vi "Callback_Roller_Fire.vi"   [LabVIEW 2011]
uses:
  roller/roller_internal_state.ctl
  roller/roller_globals.vi
types:
  T1 = typedef "roller_internal_state.ctl" = enum16{"idle", "collect", "blow", "fire_entry"}
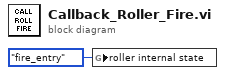
[diagram p0: block diagram]
diagram:
  n1 = global write "roller_globals.vi" "roller internal state"(roller_internal_state."fire_entry" ("roller internal state")) -> ()
